vi "Evaluate Hall Test 3.vi"(1 "String In":string) -> (0 "Test OK":bool)   [LabVIEW 2023]
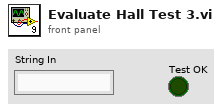
[diagram p1: front panel]
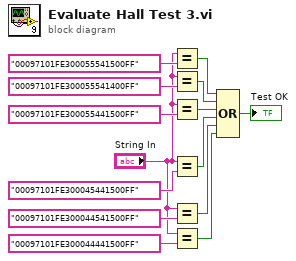
[diagram p0: block diagram]
diagram:
  n1 = Equal?(x="String In", y="00097101FE300055541500FF" ("Self Test BIST")) -> (x = y?=w6:bool)
  n2 = Equal?(x="String In", y="00097101FE300055541400FF") -> (x = y?=w5:bool)
  n3 = Equal?(x="String In", y="00097101FE300055441500FF") -> (x = y?=w4:bool)
  n4 = Equal?(x="String In", y="00097101FE300045441500FF") -> (x = y?=w7:bool)
  n5 = Equal?(x="String In", y="00097101FE300044541500FF") -> (x = y?=w8:bool)
  n6 = Equal?(x="String In", y="00097101FE300044441500FF") -> (x = y?=w1:bool)
  n7 = Compound Arithmetic op=OR(w6, w5, w4, w7, w8, w1) -> (→"Test OK":bool)
